vi "read_metadata_json.vi"(11 "Path":path) -> (0 "exp_time":string, 1 "genotype":string, 2 "fly_name":string, 3 "exp_ name":string, 6 "error out":errorcluster)   [LabVIEW 2015]
panel:
  out "JSON text":string
  # "Output from metadata file"
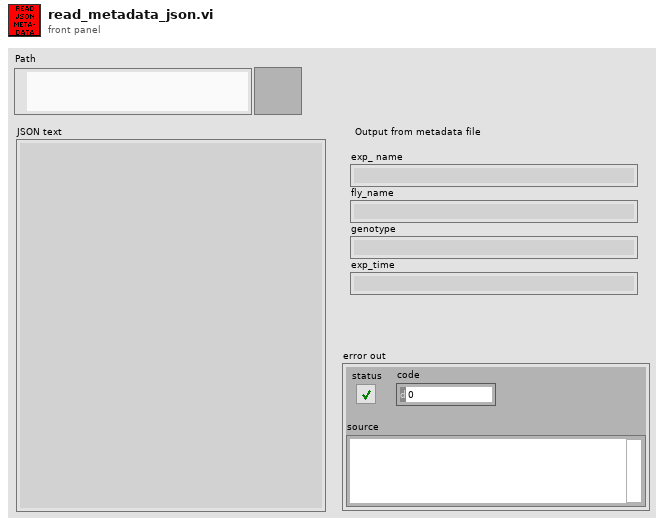
[diagram p1: front panel]
types:
  T1 = enum16{"open", "replace", "create", "open or create", "replace or create", "replace or create with confirmation"}
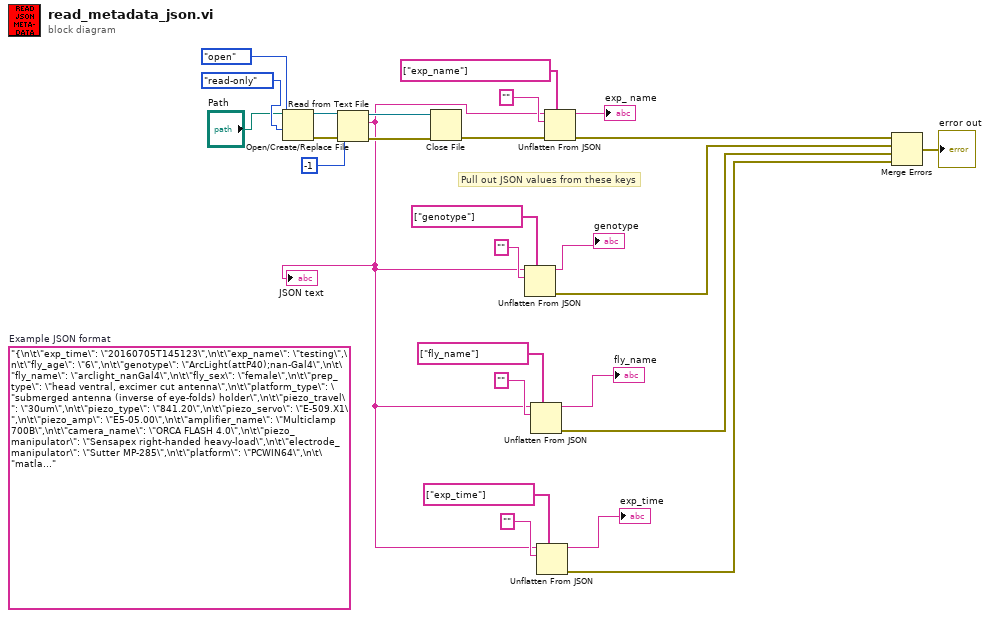
[diagram p0: block diagram]
diagram:
  (unwired) "{\n\t\"exp_time\": \"20160705T145123\",\n\t\"exp_name\": \"testing\",\n\t\"fly_age\": \"6\",\n\t\"genotype\": \"ArcLight(attP40);nan-Gal4\",\n\t\"fly_name\": \"arclight_nanGal4\",\n\t\"fly_sex\": \"female\",\n\t\"prep_type\": \"head ventral, excimer cut antenna\",\n\t\"platform_type\": \"submerged antenna (inverse of eye-folds) holder\",\n\t\"piezo_travel\": \"30um\",\n\t\"piezo_type\": \"841.20\",\n\t\"piezo_servo\": \"E-509.X1\",\n\t\"piezo_amp\": \"E5-05.00\",\n\t\"amplifier_name\": \"Multiclamp 700B\",\n\t\"camera_name\": \"ORCA FLASH 4.0\",\n\t\"piezo_manipulator\": \"Sensapex right-handed heavy-load\",\n\t\"electrode_manipulator\": \"Sutter MP-285\",\n\t\"platform\": \"PCWIN64\",\n\t\"matlab_ver\": \"9.0.0.341360 (R2016a)\"\n}"  # Example JSON format
  # "Pull out JSON values from these keys"
  n1 = Open/Create/Replace File(file path (use dialog)="Path", operation (0:open)=T1."open", access (0:read/write)=enum16{"read/write", "read-only", "write-only"}."read-only") -> (refnum out=w24:refnum<file>, error out=w23:errorcluster)  [unwired: 3 in, 1 out]
  n2 = Read from Text File(file (use dialog)=w24, count=-1, error in=w23) -> (refnum out=w26:refnum<file>, text=w2:string, error out=w25:errorcluster)  [unwired: 1 in, 1 out]
  "JSON text" <- w2
  n3 = Close File(refnum=w26, error in=w25) -> (error out=w20:errorcluster)  [unwired: 1 out]
  n4 = Unflatten From JSON(path=string[] ["genotype"], JSON string=w2, type and defaults="") -> (value=→"genotype":string, error out=w12:errorcluster)  [unwired: 4 in]
  n5 = Unflatten From JSON(path=string[] ["fly_name"], JSON string=w2, type and defaults="") -> (value=→"fly_name":string, error out=w10:errorcluster)  [unwired: 4 in]
  n6 = Unflatten From JSON(path=string[] ["exp_time"], JSON string=w2, type and defaults="") -> (value=→"exp_time":string, error out=w1:errorcluster)  [unwired: 4 in]
  n7 = Unflatten From JSON(path=string[] ["exp_name"], JSON string=w2, type and defaults="", error in (no error)=w20) -> (value=→"exp_ name":string, error out=w14:errorcluster)  [unwired: 3 in]
  n8 = Merge Errors(w14, w12, w10, w1) -> (→"error out":errorcluster)
